vi "Calculate DO Pin.vi"(0 "Row":i32, 3 "Col":i32) -> (5 "MC Pin":u8)   [LabVIEW 2017]
doc: "This VI takes the row and column indices of 3 column 2D array as input. It outputs the cell number. In the main function's application, this VI will output the pin number on microcontroller (numbered 1 -6) corresponding to the cell clicked in the 2D array."
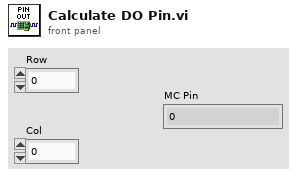
[diagram p1: front panel]
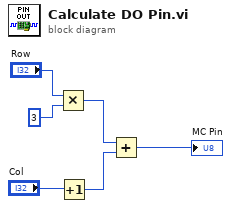
[diagram p0: block diagram]
diagram:
  n1 = Multiply(x="Row", y=3) -> (x*y=w5:i32)
  n2 = Increment(x="Col") -> (x+1=w2:i32)
  n3 = Add(x=w5, y=w2) -> (x+y=→"MC Pin":i32)
